vi "Tau start.vi"() -> ()   [LabVIEW 2019]
doc: "This global variable \"tau\" is the shared global variable set between the VIs alpha and omega.\n\nJuan Gamez\nP3600\nCSUSB Physics"
panel:
  out "Global stop":bool
  out "Active":bool
  in  "Published text":string
  in  "Published Number":dbl
  # "Alpha initializes the global variables to defaults"
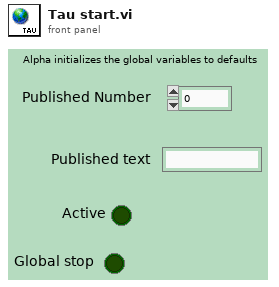
[diagram p1: front panel]
diagram:
